vi "Untitled 18 (SubVI).vi"(10 "Array in":i8[][](array[numeric]), 11 "Кол-во копий":i32) -> (3 "Array out":dbl[](array[numeric]))   [LabVIEW 2017]
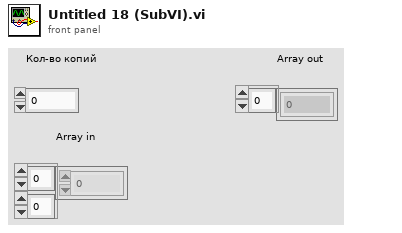
[diagram p1: front panel]
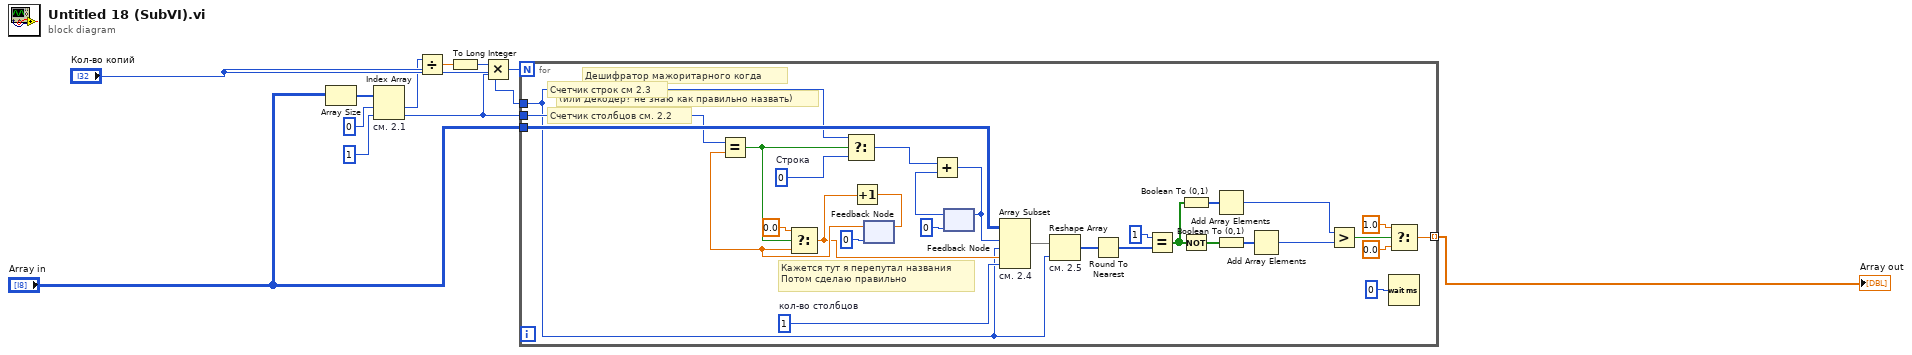
[diagram p0: block diagram]
diagram:
  # "(или Декодер? не знаю как правильно назвать)"
  # "Дешифратор мажоритарного когда"
  n1 = Array Size(array="Array in") -> (size(s)=w1:i32[])
  n2 = Index Array "см. 2.1"(array=w1, index #1=0 ("index"), index #2=1 ("index")) -> (element #1=w4:i32, element #2=w5:i32)
  n3 = Divide(x=w4, y="Кол-во копий") -> (x/y=w6:dbl)
  n4 = To Long Integer(number=w6) -> (32bit integer=w7:i32)
  n5 = Multiply(x=w7, y=w5) -> (x*y=w10:i32)
  n6 = for {
    N: w10 -> [_]
    tunnel: "Array in" -> [w40]
    tunnel: w5 -> [w32]
    tunnel: "Кол-во копий" -> [w25]
    tunnel: [w15] -> w11 mode=indexing
    w39 = 1  # кол-во столбцов
    w30 = 0  # Строка
    # "Кажется тут я перепутал названия  \nПотом сделаю правильно"
    # "Счетчик строк см 2.3"
    # "Счетчик столбцов см. 2.2"
    n7 = feedback #1(0) -> (w28:dbl)
    n8 = Equal?(x=w32, y=w28) -> (x = y?=w34:bool)
    n9 = Select(t=0.0, s=w34, f=w28) -> (s? t:f=w27:dbl)
    n10 = Select(t=w25, s=w34, f=w30) -> (s? t:f=w31:i32)
    n11 = Increment(x=w27) -> (x+1=w26:dbl)
    n12 = feedback-in #1(w26) -> ()
    n13 = feedback #2(0) -> (w33:i32)
    n14 = Add(x=w31, y=w33) -> (x+y=w29:i32)
    n15 = feedback-in #2(w29) -> ()
    n16 = Array Subset "см. 2.4"(array=w40, index (row)=w29, length (row)=w25, index (col)=w27, length (col)=w39) -> (w41:i8[][])
    n17 = Reshape Array "см. 2.5"(w41, w25) -> (w12:i8[])
    n18 = Round To Nearest(number=w12) -> (nearest integer value=w16:i8[])
    n19 = Equal?(x=1, y=w16) -> (x = y?=w18:bool[])
    n20 = Boolean To (0,1)(Boolean=w18) -> (0, 1=w14:i16[])
    n21 = Not(x=w18) -> (.not. x?=w19:bool[])
    n22 = Add Array Elements(numeric array=w14) -> (sum=w21:i16)
    n23 = Boolean To (0,1)(Boolean=w19) -> (0, 1=w13:i16[])
    n24 = Add Array Elements(numeric array=w13) -> (sum=w20:i16)
    n25 = Greater?(x=w21, y=w20) -> (0:w24:bool)
    n26 = Select(t=1.0, s=w24, f=0.0) -> (s? t:f=w15:dbl)
    n27 = Wait (ms)(milliseconds to wait=u32 0) -> ()  [unwired: 1 out]
  }
  "Array out" <- w11
